vi "SQ Lite Write Event_BW.vi"() -> ()   [LabVIEW 2017, in "Copy of Beltwatch SQLite.lvlib"]
uses:
  Beltwatch/BeltWatch 4-2-2-5/Database/Copy of Beltwatch SQLite.lvlib
  SQ Lite Cluster Action.ctl
  Beltwatch/SourceCode/BeltWatch Event.ctl
  Beltwatch/SourceCode/BeltWatch Event type.ctl
  Beltwatch/SourceCode/BeltWatch Reading.ctl
  Beltwatch/SourceCode/BeltWatch Alarm Priority.ctl
  Beltwatch/SourceCode/BeltWatch 2D overlay.ctl
  Beltwatch/SourceCode/Overlay mode.ctl
  Beltwatch/SourceCode/Events class.ctl
panel:
  out "xml string":string
  out "type string":i16[](array[numeric])
  out "?":string
  out "size(s) 2":i32
  out "size(s)":i32
  out "Controls[]":refnum<vi>[](array[refnum])
  in  "Event":T1
  out "?":errorcluster
  out "String":string
  out "SQLite3 type":T8(ring)
  in  "Event":T9[](array[typedef])=[{"Include"=TRUE, "Name"="Position", "SQLite3 type"=enum."SQLITE_INTEGER"}, {"Include"=TRUE, "Name"="Event Type", "SQLite3 type"=enum."SQLITE_INTEGER"}, {"Include"=TRUE, "Name"="Area", "SQLite3 type"=enum."SQLITE_INTEGER"}, {"Include"=TRUE, "Name"="Channels", "SQLite3 type"=enum."SQLITE_INTEGER"}, {"Include"=TRUE, "Name"="Start position", "SQLite3 type"=enum."SQLITE_INTEGER"}, {"Include"=TRUE, "Name"="End  position", "SQLite3 type"=enum."SQLITE_INTEGER"}, {"Include"=TRUE, "Name"="Name", "SQLite3 type"=enum."SQLITE3_TEXT"}, {"Include"=TRUE, "Name"="Offset", "SQLite3 type"=enum."SQLITE_INTEGER"}, {"Include"=TRUE, "Name"="Length", "SQLite3 type"=enum."SQLITE_INTEGER"}, {"Include"=TRUE, "Name"="Action marker", "SQLite3 type"=enum."SQLITE3_TEXT"}, {"Include"=TRUE, "Name"="Event", "SQLite3 type"=enum."SQLITE_INTEGER"}, {"Include"=TRUE, "Name"="# Defects", "SQLite3 type"=enum."SQLITE_INTEGER"}, {"Include"=TRUE, "Name"="jpg Image", "SQLite3 type"=enum."SQLITE_BLOB"}, {"Include"=TRUE, "Name"="chan maxs", "SQLite3 type"=enum."SQLITE_INTEGER"}, {"Include"=TRUE, "Name"="chan mins", "SQLite3 type"=enum."SQLITE_INTEGER"}, {"Include"=TRUE, "Name"="TimeStamp", "SQLite3 type"=enum."SQLITE_INTEGER"}, {"Include"=TRUE, "Name"="Readings", "SQLite3 type"=enum."SQLITE3_TEXT"}, {"Include"=TRUE, "Name"="ID", "SQLite3 type"=enum."SQLITE_INTEGER"}, {"Include"=TRUE, "Name"="New", "SQLite3 type"=enum."SQLITE_INTEGER"}, {"Include"=TRUE, "Name"="Hires Track", "SQLite3 type"=enum."SQLITE_INTEGER"}, {"Include"=TRUE, "Name"="2D overlay", "SQLite3 type"=enum."SQLITE_INTEGER"}, {"Include"=TRUE, "Name"="update", "SQLite3 type"=enum."SQLITE_INTEGER"}, {"Include"=TRUE, "Name"="Field #", "SQLite3 type"=enum."SQLITE_INTEGER"}, {"Include"=TRUE, "Name"="Events Class", "SQLite3 type"=enum."SQLITE_INTEGER"}, {"Include"=TRUE, "Name"="Sync", "SQLite3 type"=enum."SQLITE_INTEGER"}, {"Include"=TRUE, "Name"="Insert Offset", "SQLite3 type"=enum."SQLITE_INTEGER"}, {"Include"=TRUE, "Name"="Next trend", "SQLite3 type"=enum."SQLITE_INTEGER"}, {"Include"=TRUE, "Name"="Speed", "SQLite3 type"=enum."SQLITE_INTEGER"}]
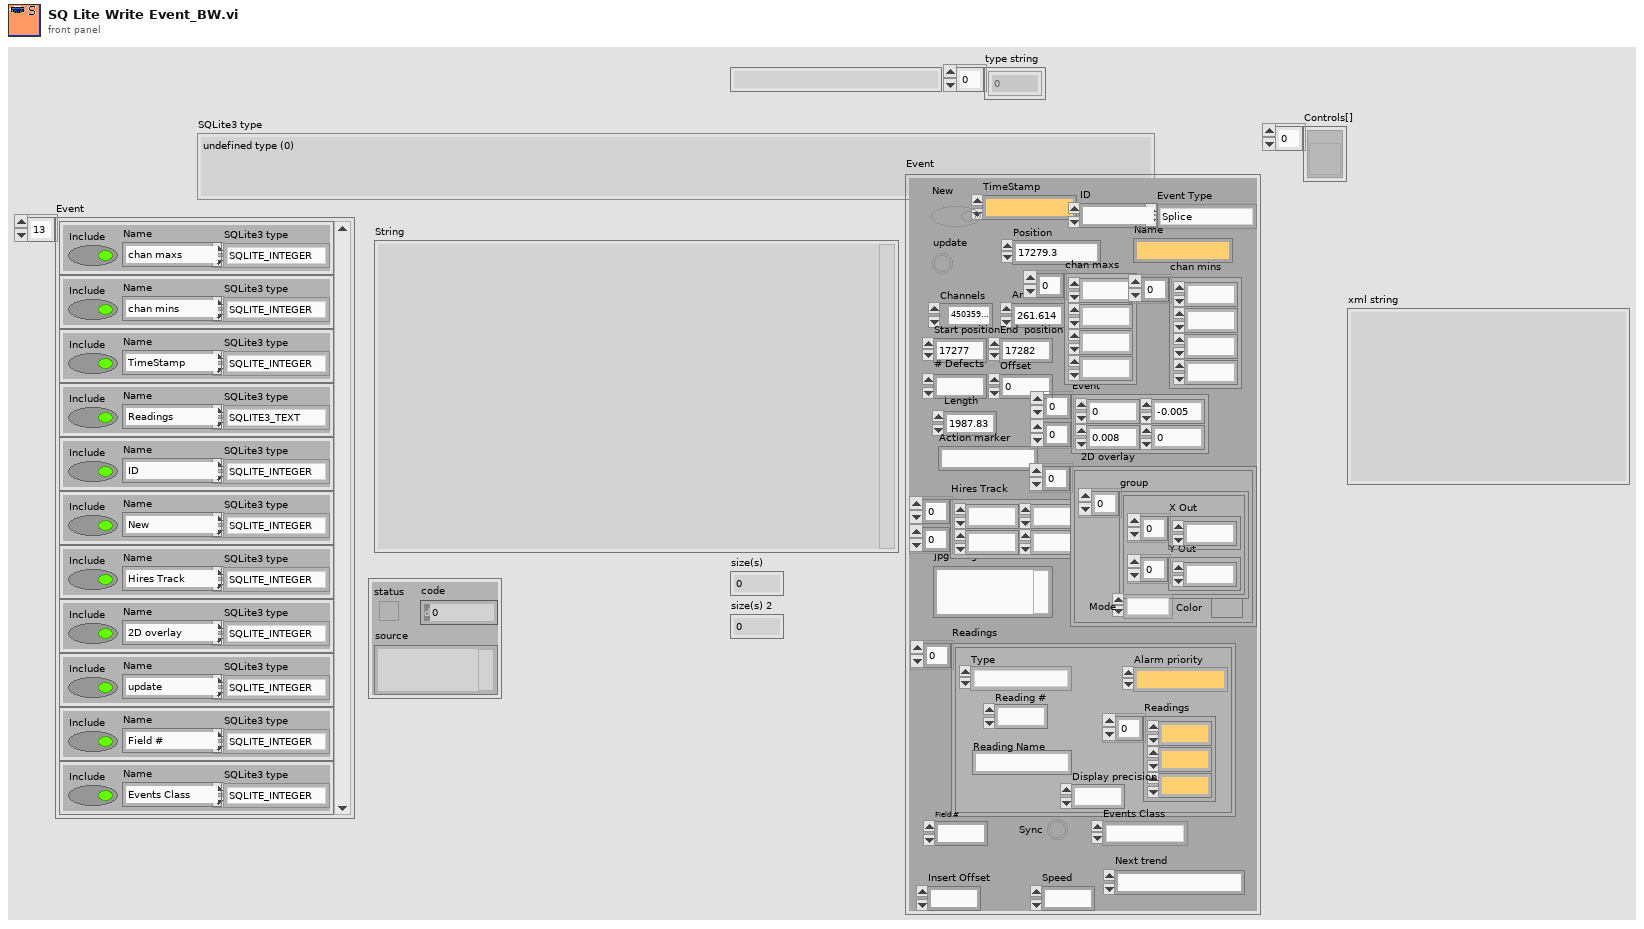
[diagram p1: front panel]
types:
  T1 = typedef "BeltWatch Event.ctl" = cluster{"Position":dbl, "Event Type":T2, "Area":dbl, "Channels":u64, "Start position":dbl, "End  position":dbl, "Name":string, "Offset":dbl, "Length":dbl, "Action marker":string, "Event":dbl[][], "# Defects":i32, "jpg Image":string, "chan maxs":dbl[], "chan mins":dbl[], "TimeStamp":dbl, "Readings":T3[], "ID":u32, "New":bool, "Hires Track":dbl[][], "2D overlay":T5, "update":bool, "Field #":i32, "Events Class":T7, "Sync":bool, "Insert Offset":dbl, "Next trend":dbl, "Speed":dbl}
  T2 = typedef "BeltWatch Event type.ctl" = enum16{"Defect", "Splice", "Break", "Rip", "Track", "Segment", "Belt", "New Splice", "Missing Splice", "None", "Free"}
  T3 = typedef "BeltWatch Reading.ctl" = cluster{"Reading #":i32, "Readings":dbl[], "Reading Name":string, "Type":T2, "Alarm priority":T4, "Display precision":i32}
  T4 = typedef "BeltWatch Alarm Priority.ctl" = enum16{"No Alarm", "High", "Medium", "Low"}
  T5 = typedef "BeltWatch 2D overlay.ctl" = cluster{"group":cluster{"X Out":sgl[], "Y Out":sgl[]}[], "Color ":u32, "Mode":T6}[]
  T6 = typedef "Overlay mode.ctl" = enum16{"Line", "point", "Box", "Oval", "Numbannotation"}
  T7 = typedef "Events class.ctl" = enum16{"Reference", "Inspection", "New", "Tramp", "Align", "Ready"}
  T8 = enum32{"undefined type (0)", "SQLITE_INTEGER", "SQLITE_FLOAT", "SQLITE3_TEXT", "SQLITE_BLOB", "SQLITE_NULL", "undefined type"}
  T9 = typedef "Copy of Beltwatch SQLite.lvlib/SQ Lite Cluster Action.ctl" = cluster{"Include":bool, "Name":string, "SQLite3 type":enum32{"undefined type (0)", "SQLITE_INTEGER", "SQLITE_FLOAT", "SQLITE3_TEXT", "SQLITE_BLOB", "SQLITE_NULL", "undefined type"}}
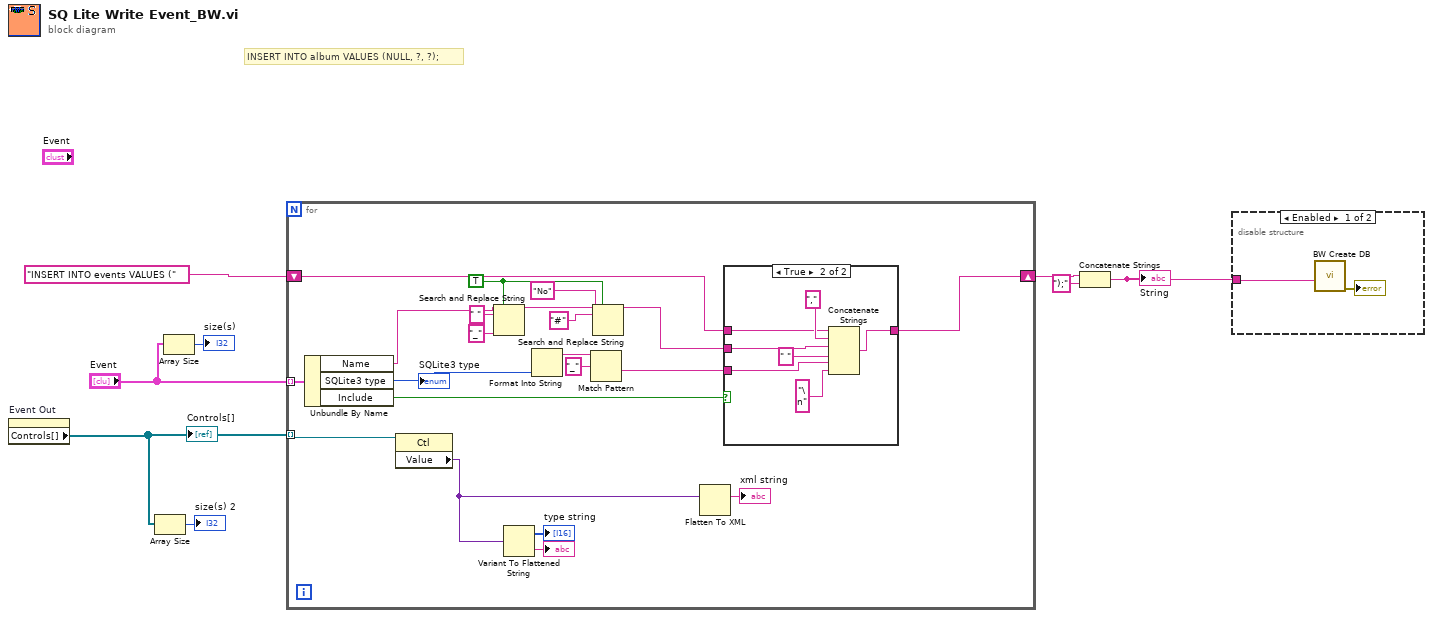
[diagram p0: block diagram]
diagram:
  # "INSERT INTO album VALUES (NULL, ?, ?);"
  n1 = property on="Event Out" class="Clust (strict)"() -> ("Controls[]"=w1:refnum<vi>[])  [unwired: 2 in, 2 out]
  "Controls[]" <- w1
  n2 = Array Size(array=w1) -> (size(s)=→"size(s) 2":i32)
  n3 = Array Size(array="Event") -> (size(s)=→"size(s)":i32)
  n4 = for {
    shift-right: [w23] -> w7
    shift-left: "INSERT INTO events VALUES (" -> [w29]
    tunnel: "Event" -> [w28] mode=indexing
    tunnel: w1 -> [w14] mode=indexing
    w19 = TRUE ("replace all? (F)")
    n5 = Unbundle By Name(w28) -> ("Name"=w22:string, "SQLite3 type"=w13:T8, "Include"=w27:bool)
    "SQLite3 type" <- w13
    n6 = property class="Ctl"(reference=w14) -> ("Value"=w10:variant)  [unwired: 1 in, 2 out]
    n7 = Search and Replace String(replace all?=w19, input string=w22, search string=" ", replace string="_" ("replace string (\"\")")) -> (result string=w18:string)  [unwired: 4 in, 3 out]
    n8 = Variant To Flattened String(Variant=w10) -> (data string=→"?":string, 1:→"type string":i16[])
    n9 = Format Into String(w13) -> (resulting string=w26:string)  [unwired: 3 in, 1 out]
    n10 = Match Pattern(string=w26, regular expression="_") -> (after substring=w24:string)  [unwired: 1 in, 3 out]
    n11 = Search and Replace String(replace all?=w19, input string=w18, search string="#" ("replace string (\"\")"), replace string="No" ("replace string (\"\")")) -> (result string=w15:string)  [unwired: 4 in, 3 out]
    n12 = Flatten To XML(anything=w10) -> (xml string=→"xml string":string)
    n13 = case shown="True" w27 {
      tunnel: w29 -> [w30 w33]
      tunnel: w15 -> [_ w37]
      tunnel: w24 -> [_ w31]
      tunnel: [w30 w35] -> w23
      frame False {
      }
      frame True {
        n14 = Concatenate Strings(w33, "," ("string"), w37, " " ("string"), w31, "\n" ("string")) -> (w35:string)
      }
    }
  }
  n15 = Concatenate Strings(w7, ");" ("string")) -> (w5:string)
  "String" <- w5
  n16 = disable-structure shown="Enabled" {
    disable-tunnel: w5 -> [w39 _]
    frame Enabled {
      n17 = call "BW Create DB.vi"("String"=w39) -> ("error out"=→"?":errorcluster)  [unwired: 10 in]
    }
    frame Disabled {
    }
  }
